vi "input.vi"(8 "error in":errorcluster, 10 "data table in":T1, 11 "FPGA Module runtime in":refnum<class "FPGA Module runtime.lvclass">) -> (0 "error out":errorcluster, 2 "data table out":T1, 3 "FPGA Module runtime out":refnum<class "FPGA Module runtime.lvclass">)   [LabVIEW 2014, in "FPGA Module runtime.lvclass"]
doc: "Provides an interface for reading data from a module at runtime. While this interface performs no operations, a child should provide an override which may read from any open sessions, references, or interfaces."
uses:
  FPGA Module runtime.lvclass
  <vilib>/NI/Tag Bus/table/data table.ctl
  FPGA Module runtime.lvclass/FPGA Module runtime.ctl
  OLD Project Folder/fpga channel/FXP I_20_5.ctl
  OLD Project Folder/fpga channel/FXP I_24_5.ctl
  OLD Project Folder/fpga channel/FXP I_24_10.ctl
  <vilib>/NI/Tag Bus/table/data polymorphs/write many/write Doubles.vi
  <vilib>/NI/Tag Bus/table/data polymorphs/write many/write Singles.vi
  <vilib>/NI/Tag Bus/table/data polymorphs/write many/write I64s.vi
  <vilib>/NI/Tag Bus/table/data polymorphs/write many/write I32s.vi
  <vilib>/NI/Tag Bus/table/data polymorphs/write many/write I16s.vi
  <vilib>/NI/Tag Bus/table/data polymorphs/write many/write I8s.vi
  <vilib>/NI/Tag Bus/table/data polymorphs/write many/write U64s.vi
  <vilib>/NI/Tag Bus/table/data polymorphs/write many/write U32s.vi
  <vilib>/NI/Tag Bus/table/data polymorphs/write many/write U16s.vi
  <vilib>/NI/Tag Bus/table/data polymorphs/write many/write U8s.vi
  <vilib>/NI/Tag Bus/table/data polymorphs/write many/write Booleans.vi
  <vilib>/NI/Tag Bus/table/data polymorphs/write one/write Array of Single.vi
  <vilib>/NI/Tag Bus/table/data polymorphs/write one/write Array of I64.vi
  <vilib>/NI/Tag Bus/table/data polymorphs/write one/write Array of I32.vi
  <vilib>/NI/Tag Bus/table/data polymorphs/write one/write Array of I16.vi
  <vilib>/NI/Tag Bus/table/data polymorphs/write one/write Array of I8.vi
  <vilib>/NI/Tag Bus/table/data polymorphs/write one/write Array of U64.vi
  <vilib>/NI/Tag Bus/table/data polymorphs/write one/write Array of U32.vi
  <vilib>/NI/Tag Bus/table/data polymorphs/write one/write Array of U16.vi
  <vilib>/NI/Tag Bus/table/data polymorphs/write one/write Array of U8.vi
  <vilib>/NI/Tag Bus/table/data polymorphs/write one/write Array of Boolean.vi
  <vilib>/rvi/errors/niLvFpgaAdjustHostInterfaceError.vi
  <vilib>/Utility/error.llb/Error Cluster From Error Code.vi
  <vilib>/rvi/interface/nirviReadWriteControl/nirviReadWriteControl.xnode
  <vilib>/NI/Tag Bus/table/data table.lvlib
  fpga channel/FPGA Channel.lvclass
  NiFpgaLv.dll
  <vilib>/rvi/interface/Simulation/niFpgaSimulationCallBeginRW.vi
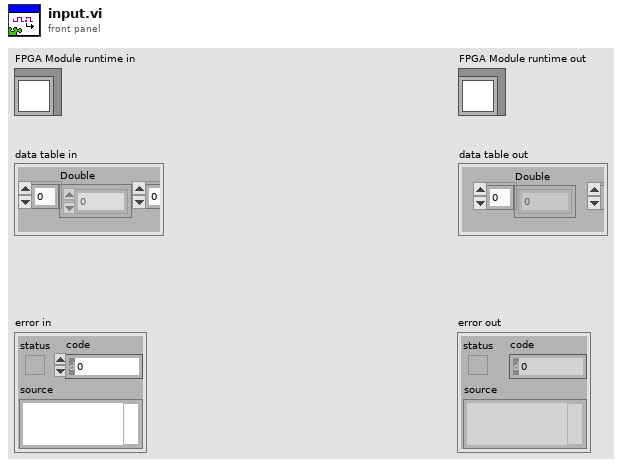
[diagram p1: front panel]
types:
  T1 = typedef "tag bus.lvlib/data table.lvlib/data table.ctl" = cluster{"Double":dbl[], "Single":sgl[], "I64":i64[], "I32":i32[], "I16":i16[], "I8":i8[], "U64":u64[], "U32":u32[], "U16":u16[], "U8":u8[], "Boolean":bool[], "String":string[], "Array of Double":cluster{"DBL Array":dbl[]}[], "Array of Single":cluster{"SGL Array":sgl[]}[], "Array of I64":cluster{"I64 Array":i64[]}[], "Array of I32":cluster{"I32 Array":i32[]}[], "Array of I16":cluster{"I16 Array":i16[]}[], "Array of I8":cluster{"I8 Array":i8[]}[], "Array of U64":cluster{"U64 Array":u64[]}[], "Array of U32":cluster{"U32 Array":u32[]}[], "Array of U16":cluster{"U16 Array":u16[]}[], "Array of U8":cluster{"U8 Array":u8[]}[], "Array of Boolean":cluster{"Boolean Array":bool[]}[], "Array of String":cluster{"String Array":string[]}[]}
  T2 = typedef "FPGA Module runtime.lvclass/ControlsMappings.ctl" = cluster{"data type":T3, "fpga res type":T4[], "fpga resource":refnum<k20>[], "data indexes":i32[]}
  T3 = typedef "tag bus.lvlib/tag descriptor.lvclass/Data Type.ctl" = enum16{"Double", "Single", "I64", "I32", "I16", "I8", "U64", "U32", "U16", "U8", "Boolean", "String", "Array of Double", "Array of Single", "Array of I64", "Array of I32", "Array of I16", "Array of I8", "Array of U64", "Array of U32", "Array of U16", "Array of U8", "Array of Boolean", "Array of String"}
  T4 = typedef "FPGA Channel.lvclass/fpga resource supported data types.ctl" = enum16{"Invalid Type", "Single", "I64", "I32", "I16", "I8", "U64", "U32", "U16", "U8", "Boolean", "FXP I,20,5", "FXP I,24,5", "FXP I,24,10", "Fifo 1023,I16"}
  T5 = typedef "FPGA Channel.lvclass/FXP I_20_5.ctl" = refnum<k20>
  T6 = typedef "FPGA Channel.lvclass/FXP I_24_5.ctl" = refnum<k20>
  T7 = typedef "FPGA Channel.lvclass/FXP I_24_10.ctl" = refnum<k20>
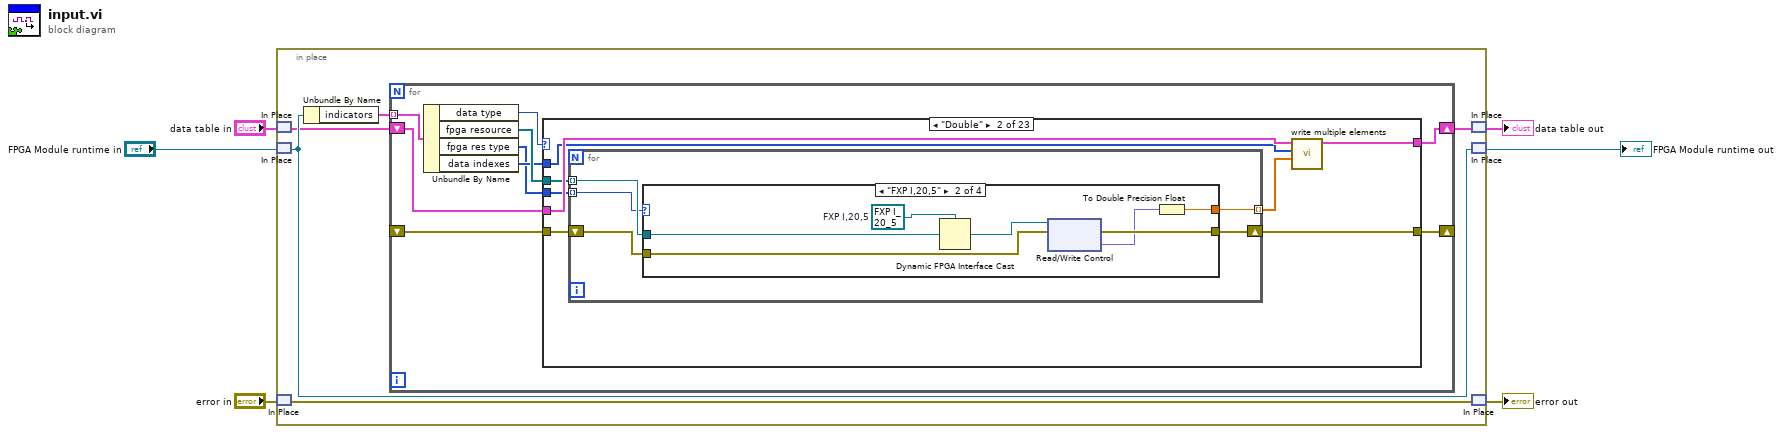
[diagram p0: block diagram]
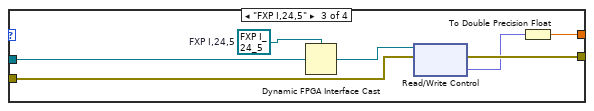
[diagram p4: hidden frame]
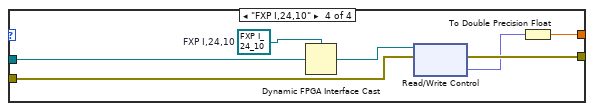
[diagram p5: hidden frame]
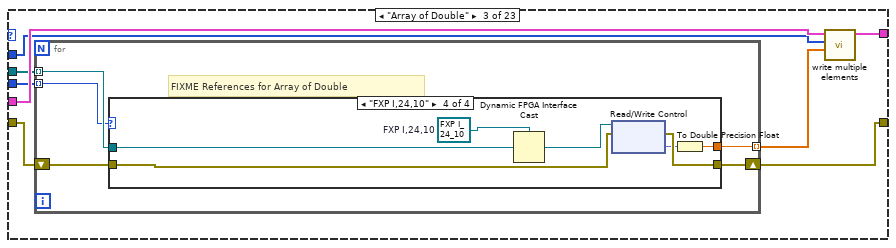
[diagram p6: hidden frame]
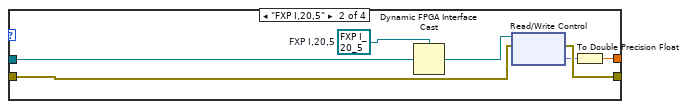
[diagram p8: hidden frame]
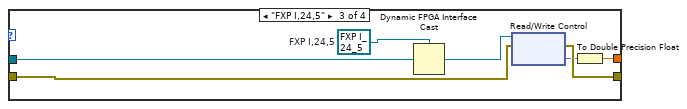
[diagram p9: hidden frame]
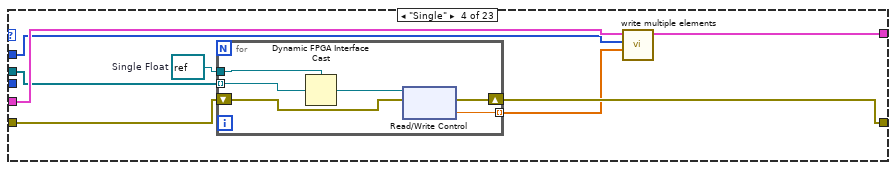
[diagram p10: hidden frame]
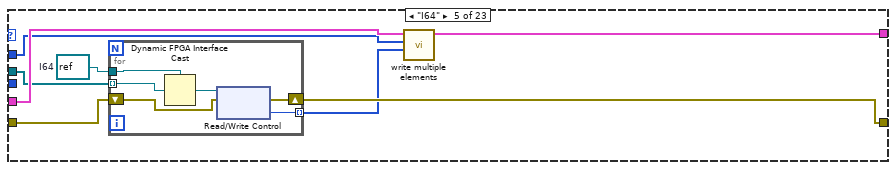
[diagram p11: hidden frame]
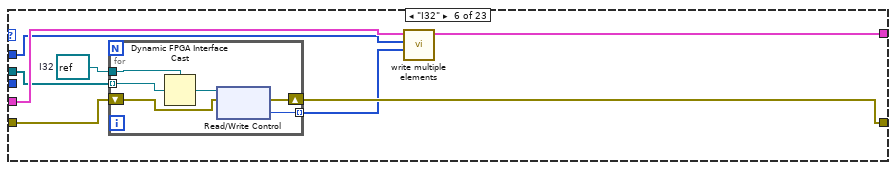
[diagram p12: hidden frame]
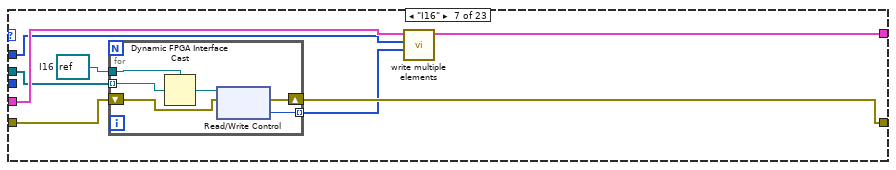
[diagram p13: hidden frame]
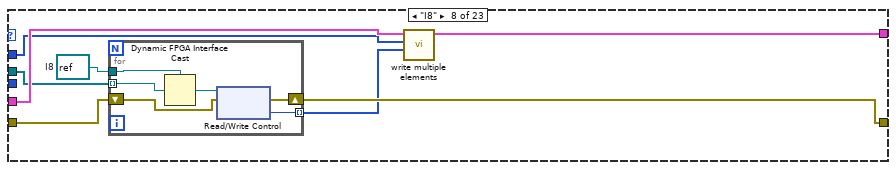
[diagram p14: hidden frame]
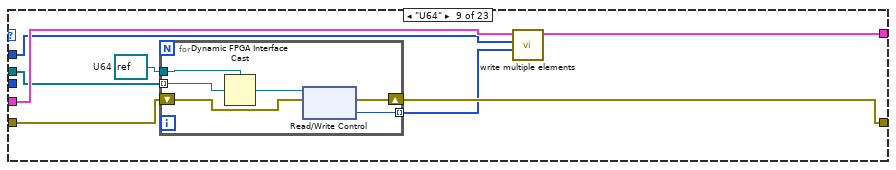
[diagram p15: hidden frame]
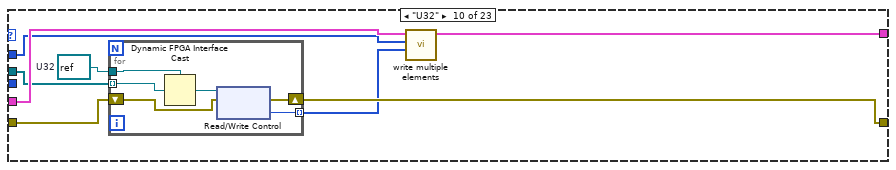
[diagram p16: hidden frame]
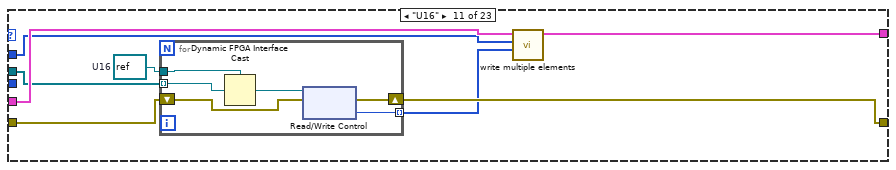
[diagram p17: hidden frame]
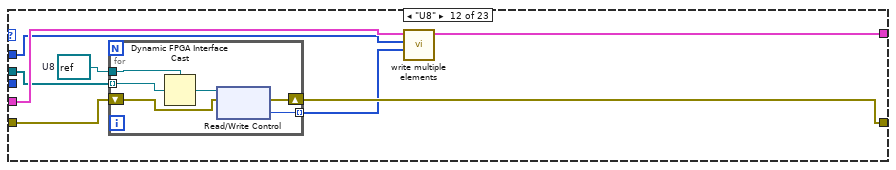
[diagram p18: hidden frame]
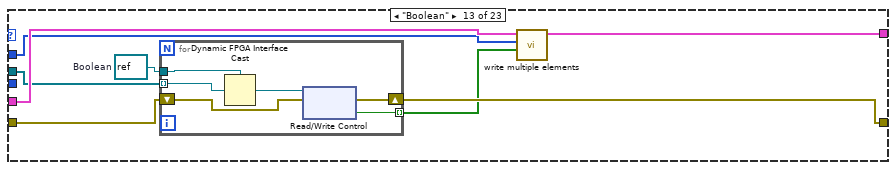
[diagram p19: hidden frame]
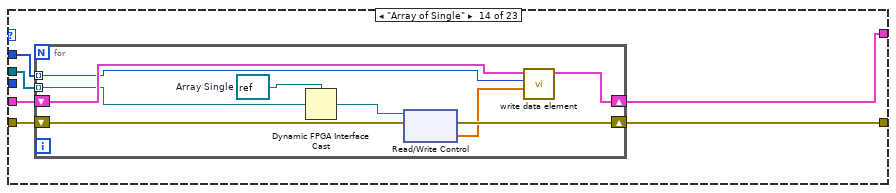
[diagram p20: hidden frame]
diagram:
  n1 = in-place {
    n2 = in-place-match #1("data table in") -> (w7:T1)
    n3 = in-place-match #2("FPGA Module runtime in") -> (w10:refnum<class "FPGA Module runtime.lvclass">)
    n4 = in-place-match #3("error in") -> (w11:errorcluster)
    n5 = Unbundle By Name(w10) -> ("indicators"=w8:T2[])
    n6 = for {
      shift-right: [w17] -> w9
      shift-left: w7 -> [w18]
      shift-right: [w16] -> _
      shift-left: _ -> [w15]
      tunnel: w8 -> [w20] mode=indexing
      n7 = Unbundle By Name(w20) -> ("data type"=w19:T3, "fpga resource"=w14:refnum<k20>[], "fpga res type"=w12:T4[], "data indexes"=w13:i32[])
      n8 = case shown="\"Double\"" w19 {
        tunnel: w13 -> [_ w23 w58 w98 w111 w126 w140 w154 w168 w182 w196 w210 w224 w236 w251 w266 w281 w296 w311 w326 w341 w356 w371]
        tunnel: w15 -> [w22 w27 w62 w96 w114 w124 w138 w152 w166 w180 w194 w208 w222 w235 w250 w265 w280 w295 w310 w325 w340 w355 w370]
        tunnel: w18 -> [w21 w30 w65 w100 w113 w128 w142 w156 w170 w184 w198 w212 w226 w238 w253 w268 w283 w298 w313 w328 w343 w358 w373]
        tunnel: [w21 w29 w64 w99 w112 w127 w141 w155 w169 w183 w197 w211 w225 w237 w252 w267 w282 w297 w312 w327 w342 w357 w372] -> w17
        tunnel: [w22 w26 w61 w95 w109 w123 w137 w151 w165 w179 w193 w207 w221 w234 w249 w264 w279 w294 w309 w324 w339 w354 w369] -> w16
        tunnel: w14 -> [_ w28 w63 w97 w110 w125 w139 w153 w167 w181 w195 w209 w223 w233 w248 w263 w278 w293 w308 w323 w338 w353 w368]
        tunnel: w12 -> [_ w25 w60 _ _ _ _ _ _ _ _ _ _ _ _ _ _ _ _ _ _ _ _]
        frame Default {
        }
        frame "Double" {
          n9 = for {
            tunnel: w28 -> [w35] mode=indexing
            shift-right: [w33] -> w26
            shift-left: w27 -> [w34]
            tunnel: [w32] -> w24 mode=indexing
            tunnel: w25 -> [w31] mode=indexing
            n10 = case shown="\"FXP I,20,5\"" w31 {
              tunnel: w35 -> [_ w43 w50 w57]
              tunnel: w34 -> [w36 w42 w49 w56]
              tunnel: [w36 w41 w48 w55] -> w33
              tunnel: [_ w38 w45 w52] -> w32
              frame "Invalid Type", Default {
              }
              frame "FXP I,20,5" {
                w40 = T5 refnum  # FXP I,20,5
                n11 = Dynamic FPGA Interface Cast(Session In=w40, Type=w43) -> (Session Out=w37:T5)
                n12 = xnode "Read/Write Control"("FPGA VI Reference In"=w37, "error in"=w42) -> ("error out"=w41:errorcluster, "Value"=w39:fxp<+/-,20,5>)  [unwired: 1 out]
                n13 = To Double Precision Float(number=w39) -> (double precision float=w38:dbl)
              }
              frame "FXP I,24,5" {
                w47 = T6 refnum  # FXP I,24,5
                n14 = Dynamic FPGA Interface Cast(Session In=w47, Type=w50) -> (Session Out=w44:T6)
                n15 = xnode "Read/Write Control"("FPGA VI Reference In"=w44, "error in"=w49) -> ("error out"=w48:errorcluster, "Value"=w46:fxp<+/-,24,5>)  [unwired: 1 out]
                n16 = To Double Precision Float(number=w46) -> (double precision float=w45:dbl)
              }
              frame "FXP I,24,10" {
                w54 = T7 refnum  # FXP I,24,10
                n17 = Dynamic FPGA Interface Cast(Session In=w54, Type=w57) -> (Session Out=w51:T7)
                n18 = xnode "Read/Write Control"("FPGA VI Reference In"=w51, "error in"=w56) -> ("error out"=w55:errorcluster, "Value"=w53:fxp<+/-,24,10>)  [unwired: 1 out]
                n19 = To Double Precision Float(number=w53) -> (double precision float=w52:dbl)
              }
            }
          }
          n20 = call-poly <vilib>:"write multiple elements.vi"("values"=w24, "indices"=w23, "data table in"=w30) -> ("data table out"=w29:T1)  [unwired: 8 in]
        }
        frame "Array of Double" {
          n21 = for {
            tunnel: w63 -> [w70] mode=indexing
            shift-right: [w68] -> w61
            shift-left: w62 -> [w69]
            tunnel: [w67] -> w59 mode=indexing
            tunnel: w60 -> [w66] mode=indexing
            # "FIXME References for Array of Double"
            n22 = case shown="\"FXP I,24,10\"" w66 {
              tunnel: w70 -> [_ w78 w85 w92]
              tunnel: w69 -> [w71 w77 w84 w91]
              tunnel: [w71 w76 w83 w90] -> w68
              tunnel: [_ w73 w80 w87] -> w67
              frame "Invalid Type", Default {
              }
              frame "FXP I,20,5" {
                w75 = T5 refnum  # FXP I,20,5
                n23 = Dynamic FPGA Interface Cast(Session In=w75, Type=w78) -> (Session Out=w72:T5)
                n24 = xnode "Read/Write Control"("FPGA VI Reference In"=w72, "error in"=w77) -> ("error out"=w76:errorcluster, "Value"=w74:fxp<+/-,20,5>)  [unwired: 1 out]
                n25 = To Double Precision Float(number=w74) -> (double precision float=w73:dbl)
              }
              frame "FXP I,24,5" {
                w82 = T6 refnum  # FXP I,24,5
                n26 = Dynamic FPGA Interface Cast(Session In=w82, Type=w85) -> (Session Out=w79:T6)
                n27 = xnode "Read/Write Control"("FPGA VI Reference In"=w79, "error in"=w84) -> ("error out"=w83:errorcluster, "Value"=w81:fxp<+/-,24,5>)  [unwired: 1 out]
                n28 = To Double Precision Float(number=w81) -> (double precision float=w80:dbl)
              }
              frame "FXP I,24,10" {
                w89 = T7 refnum  # FXP I,24,10
                n29 = Dynamic FPGA Interface Cast(Session In=w89, Type=w92) -> (Session Out=w86:T7)
                n30 = xnode "Read/Write Control"("FPGA VI Reference In"=w86, "error in"=w91) -> ("error out"=w90:errorcluster, "Value"=w88:fxp<+/-,24,10>)  [unwired: 1 out]
                n31 = To Double Precision Float(number=w88) -> (double precision float=w87:dbl)
              }
            }
          }
          n32 = call-poly <vilib>:"write multiple elements.vi"("values"=w59, "indices"=w58, "data table in"=w65) -> ("data table out"=w64:T1)  [unwired: 8 in]
        }
        frame "Single" {
          w94 = refnum<k20> refnum  # Single Float
          n33 = for {
            tunnel: w97 -> [w106] mode=indexing
            shift-right: [w103] -> w95
            shift-left: w96 -> [w104]
            tunnel: [w102] -> w93 mode=indexing
            tunnel: w94 -> [w101]
            n34 = Dynamic FPGA Interface Cast(Session In=w101, Type=w106) -> (Session Out=w105:refnum<k20>)
            n35 = xnode "Read/Write Control"("FPGA VI Reference In"=w105, "error in"=w104) -> ("error out"=w103:errorcluster, "Value"=w102:sgl)  [unwired: 1 out]
          }
          n36 = call-poly <vilib>:"write multiple elements.vi"("values"=w93, "indices"=w98, "data table in"=w100) -> ("data table out"=w99:T1)  [unwired: 8 in]
        }
        frame "I64" {
          w107 = refnum<k20> refnum  # I64
          n37 = for {
            tunnel: w110 -> [w120] mode=indexing
            shift-right: [w117] -> w109
            shift-left: w114 -> [w118]
            tunnel: [w116] -> w108 mode=indexing
            tunnel: w107 -> [w115]
            n38 = Dynamic FPGA Interface Cast(Session In=w115, Type=w120) -> (Session Out=w119:refnum<k20>)
            n39 = xnode "Read/Write Control"("FPGA VI Reference In"=w119, "error in"=w118) -> ("error out"=w117:errorcluster, "Value"=w116:i64)  [unwired: 1 out]
          }
          n40 = call-poly <vilib>:"write multiple elements.vi"("values"=w108, "indices"=w111, "data table in"=w113) -> ("data table out"=w112:T1)  [unwired: 8 in]
        }
        frame "I32" {
          w121 = refnum<k20> refnum  # I32
          n41 = for {
            tunnel: w125 -> [w134] mode=indexing
            shift-right: [w131] -> w123
            shift-left: w124 -> [w132]
            tunnel: [w130] -> w122 mode=indexing
            tunnel: w121 -> [w129]
            n42 = Dynamic FPGA Interface Cast(Session In=w129, Type=w134) -> (Session Out=w133:refnum<k20>)
            n43 = xnode "Read/Write Control"("FPGA VI Reference In"=w133, "error in"=w132) -> ("error out"=w131:errorcluster, "Value"=w130:i32)  [unwired: 1 out]
          }
          n44 = call-poly <vilib>:"write multiple elements.vi"("values"=w122, "indices"=w126, "data table in"=w128) -> ("data table out"=w127:T1)  [unwired: 8 in]
        }
        frame "I16" {
          w135 = refnum<k20> refnum  # I16
          n45 = for {
            tunnel: w139 -> [w148] mode=indexing
            shift-right: [w145] -> w137
            shift-left: w138 -> [w146]
            tunnel: [w144] -> w136 mode=indexing
            tunnel: w135 -> [w143]
            n46 = Dynamic FPGA Interface Cast(Session In=w143, Type=w148) -> (Session Out=w147:refnum<k20>)
            n47 = xnode "Read/Write Control"("FPGA VI Reference In"=w147, "error in"=w146) -> ("error out"=w145:errorcluster, "Value"=w144:i16)  [unwired: 1 out]
          }
          n48 = call-poly <vilib>:"write multiple elements.vi"("values"=w136, "indices"=w140, "data table in"=w142) -> ("data table out"=w141:T1)  [unwired: 8 in]
        }
        frame "I8" {
          w149 = refnum<k20> refnum  # I8
          n49 = for {
            tunnel: w153 -> [w162] mode=indexing
            shift-right: [w159] -> w151
            shift-left: w152 -> [w160]
            tunnel: [w158] -> w150 mode=indexing
            tunnel: w149 -> [w157]
            n50 = Dynamic FPGA Interface Cast(Session In=w157, Type=w162) -> (Session Out=w161:refnum<k20>)
            n51 = xnode "Read/Write Control"("FPGA VI Reference In"=w161, "error in"=w160) -> ("error out"=w159:errorcluster, "Value"=w158:i8)  [unwired: 1 out]
          }
          n52 = call-poly <vilib>:"write multiple elements.vi"("values"=w150, "indices"=w154, "data table in"=w156) -> ("data table out"=w155:T1)  [unwired: 8 in]
        }
        frame "U64" {
          w163 = refnum<k20> refnum  # U64
          n53 = for {
            tunnel: w167 -> [w176] mode=indexing
            shift-right: [w173] -> w165
            shift-left: w166 -> [w174]
            tunnel: [w172] -> w164 mode=indexing
            tunnel: w163 -> [w171]
            n54 = Dynamic FPGA Interface Cast(Session In=w171, Type=w176) -> (Session Out=w175:refnum<k20>)
            n55 = xnode "Read/Write Control"("FPGA VI Reference In"=w175, "error in"=w174) -> ("error out"=w173:errorcluster, "Value"=w172:u64)  [unwired: 1 out]
          }
          n56 = call-poly <vilib>:"write multiple elements.vi"("values"=w164, "indices"=w168, "data table in"=w170) -> ("data table out"=w169:T1)  [unwired: 8 in]
        }
        frame "U32" {
          w177 = refnum<k20> refnum  # U32
          n57 = for {
            tunnel: w181 -> [w190] mode=indexing
            shift-right: [w187] -> w179
            shift-left: w180 -> [w188]
            tunnel: [w186] -> w178 mode=indexing
            tunnel: w177 -> [w185]
            n58 = Dynamic FPGA Interface Cast(Session In=w185, Type=w190) -> (Session Out=w189:refnum<k20>)
            n59 = xnode "Read/Write Control"("FPGA VI Reference In"=w189, "error in"=w188) -> ("error out"=w187:errorcluster, "Value"=w186:u32)  [unwired: 1 out]
          }
          n60 = call-poly <vilib>:"write multiple elements.vi"("values"=w178, "indices"=w182, "data table in"=w184) -> ("data table out"=w183:T1)  [unwired: 8 in]
        }
        frame "U16" {
          w191 = refnum<k20> refnum  # U16
          n61 = for {
            tunnel: w195 -> [w204] mode=indexing
            shift-right: [w201] -> w193
            shift-left: w194 -> [w202]
            tunnel: [w200] -> w192 mode=indexing
            tunnel: w191 -> [w199]
            n62 = Dynamic FPGA Interface Cast(Session In=w199, Type=w204) -> (Session Out=w203:refnum<k20>)
            n63 = xnode "Read/Write Control"("FPGA VI Reference In"=w203, "error in"=w202) -> ("error out"=w201:errorcluster, "Value"=w200:u16)  [unwired: 1 out]
          }
          n64 = call-poly <vilib>:"write multiple elements.vi"("values"=w192, "indices"=w196, "data table in"=w198) -> ("data table out"=w197:T1)  [unwired: 8 in]
        }
        frame "U8" {
          w205 = refnum<k20> refnum  # U8
          n65 = for {
            tunnel: w209 -> [w218] mode=indexing
            shift-right: [w215] -> w207
            shift-left: w208 -> [w216]
            tunnel: [w214] -> w206 mode=indexing
            tunnel: w205 -> [w213]
            n66 = Dynamic FPGA Interface Cast(Session In=w213, Type=w218) -> (Session Out=w217:refnum<k20>)
            n67 = xnode "Read/Write Control"("FPGA VI Reference In"=w217, "error in"=w216) -> ("error out"=w215:errorcluster, "Value"=w214:u8)  [unwired: 1 out]
          }
          n68 = call-poly <vilib>:"write multiple elements.vi"("values"=w206, "indices"=w210, "data table in"=w212) -> ("data table out"=w211:T1)  [unwired: 8 in]
        }
        frame "Boolean" {
          w219 = refnum<k20> refnum  # Boolean
          n69 = for {
            tunnel: w223 -> [w232] mode=indexing
            shift-right: [w229] -> w221
            shift-left: w222 -> [w230]
            tunnel: [w228] -> w220 mode=indexing
            tunnel: w219 -> [w227]
            n70 = Dynamic FPGA Interface Cast(Session In=w227, Type=w232) -> (Session Out=w231:refnum<k20>)
            n71 = xnode "Read/Write Control"("FPGA VI Reference In"=w231, "error in"=w230) -> ("error out"=w229:errorcluster, "Value"=w228:bool)  [unwired: 1 out]
          }
          n72 = call-poly <vilib>:"write multiple elements.vi"("values"=w220, "indices"=w224, "data table in"=w226) -> ("data table out"=w225:T1)  [unwired: 8 in]
        }
        frame "Array of Single" {
          n73 = for {
            tunnel: w236 -> [w245] mode=indexing
            shift-right: [w242] -> w234
            shift-left: w235 -> [w241]
            shift-right: [w246] -> w237
            shift-left: w238 -> [w247]
            tunnel: w233 -> [w243] mode=indexing
            w240 = refnum<k20> refnum  # Array Single
            n74 = Dynamic FPGA Interface Cast(Session In=w240, Type=w243) -> (Session Out=w244:refnum<k20>)
            n75 = xnode "Read/Write Control"("FPGA VI Reference In"=w244, "error in"=w241) -> ("error out"=w242:errorcluster, "Value"=w239:sgl[])  [unwired: 1 out]
            n76 = call-poly <vilib>:"write data element.vi"("value"=w239, "index"=w245, "data table in"=w247) -> ("data table out"=w246:T1)  [unwired: 8 in]
          }
        }
        frame "Array of I64" {
          n77 = for {
            tunnel: w251 -> [w260] mode=indexing
            shift-right: [w257] -> w249
            shift-left: w250 -> [w256]
            shift-right: [w261] -> w252
            shift-left: w253 -> [w262]
            tunnel: w248 -> [w258] mode=indexing
            w254 = refnum<k20> refnum  # Array I64
            n78 = Dynamic FPGA Interface Cast(Session In=w254, Type=w258) -> (Session Out=w259:refnum<k20>)
            n79 = xnode "Read/Write Control"("FPGA VI Reference In"=w259, "error in"=w256) -> ("error out"=w257:errorcluster, "Value"=w255:i64[])  [unwired: 1 out]
            n80 = call-poly <vilib>:"write data element.vi"("value"=w255, "index"=w260, "data table in"=w262) -> ("data table out"=w261:T1)  [unwired: 8 in]
          }
        }
        frame "Array of I32" {
          n81 = for {
            tunnel: w266 -> [w275] mode=indexing
            shift-right: [w272] -> w264
            shift-left: w265 -> [w271]
            shift-right: [w276] -> w267
            shift-left: w268 -> [w277]
            tunnel: w263 -> [w273] mode=indexing
            w269 = refnum<k20> refnum  # Array I32
            n82 = Dynamic FPGA Interface Cast(Session In=w269, Type=w273) -> (Session Out=w274:refnum<k20>)
            n83 = xnode "Read/Write Control"("FPGA VI Reference In"=w274, "error in"=w271) -> ("error out"=w272:errorcluster, "Value"=w270:i32[])  [unwired: 1 out]
            n84 = call-poly <vilib>:"write data element.vi"("value"=w270, "index"=w275, "data table in"=w277) -> ("data table out"=w276:T1)  [unwired: 8 in]
          }
        }
        frame "Array of I16" {
          n85 = for {
            tunnel: w281 -> [w290] mode=indexing
            shift-right: [w287] -> w279
            shift-left: w280 -> [w286]
            shift-right: [w291] -> w282
            shift-left: w283 -> [w292]
            tunnel: w278 -> [w288] mode=indexing
            w284 = refnum<k20> refnum  # Array I16
            n86 = Dynamic FPGA Interface Cast(Session In=w284, Type=w288) -> (Session Out=w289:refnum<k20>)
            n87 = xnode "Read/Write Control"("FPGA VI Reference In"=w289, "error in"=w286) -> ("error out"=w287:errorcluster, "Value"=w285:i16[])  [unwired: 1 out]
            n88 = call-poly <vilib>:"write data element.vi"("value"=w285, "index"=w290, "data table in"=w292) -> ("data table out"=w291:T1)  [unwired: 8 in]
          }
        }
        frame "Array of I8" {
          n89 = for {
            tunnel: w296 -> [w305] mode=indexing
            shift-right: [w302] -> w294
            shift-left: w295 -> [w301]
            shift-right: [w306] -> w297
            shift-left: w298 -> [w307]
            tunnel: w293 -> [w303] mode=indexing
            w299 = refnum<k20> refnum  # Array I8
            n90 = Dynamic FPGA Interface Cast(Session In=w299, Type=w303) -> (Session Out=w304:refnum<k20>)
            n91 = xnode "Read/Write Control"("FPGA VI Reference In"=w304, "error in"=w301) -> ("error out"=w302:errorcluster, "Value"=w300:i8[])  [unwired: 1 out]
            n92 = call-poly <vilib>:"write data element.vi"("value"=w300, "index"=w305, "data table in"=w307) -> ("data table out"=w306:T1)  [unwired: 8 in]
          }
        }
        frame "Array of U64" {
          n93 = for {
            tunnel: w311 -> [w320] mode=indexing
            shift-right: [w317] -> w309
            shift-left: w310 -> [w316]
            shift-right: [w321] -> w312
            shift-left: w313 -> [w322]
            tunnel: w308 -> [w318] mode=indexing
            n94 = Dynamic FPGA Interface Cast(Session In=refnum<k20> refnum ("FPGA VI Reference Out"), Type=w318) -> (Session Out=w319:refnum<k20>)
            n95 = xnode "Read/Write Control"("FPGA VI Reference In"=w319, "error in"=w316) -> ("error out"=w317:errorcluster, "Value"=w315:u64[])  [unwired: 1 out]
            n96 = call-poly <vilib>:"write data element.vi"("value"=w315, "index"=w320, "data table in"=w322) -> ("data table out"=w321:T1)  [unwired: 8 in]
          }
        }
        frame "Array of U32" {
          n97 = for {
            tunnel: w326 -> [w335] mode=indexing
            shift-right: [w332] -> w324
            shift-left: w325 -> [w331]
            shift-right: [w336] -> w327
            shift-left: w328 -> [w337]
            tunnel: w323 -> [w333] mode=indexing
            w329 = refnum<k20> refnum  # Array U32
            n98 = Dynamic FPGA Interface Cast(Session In=w329, Type=w333) -> (Session Out=w334:refnum<k20>)
            n99 = xnode "Read/Write Control"("FPGA VI Reference In"=w334, "error in"=w331) -> ("error out"=w332:errorcluster, "Value"=w330:u32[])  [unwired: 1 out]
            n100 = call-poly <vilib>:"write data element.vi"("value"=w330, "index"=w335, "data table in"=w337) -> ("data table out"=w336:T1)  [unwired: 8 in]
          }
        }
        frame "Array of U16" {
          n101 = for {
            tunnel: w341 -> [w350] mode=indexing
            shift-right: [w347] -> w339
            shift-left: w340 -> [w346]
            shift-right: [w351] -> w342
            shift-left: w343 -> [w352]
            tunnel: w338 -> [w348] mode=indexing
            w344 = refnum<k20> refnum  # Array U16
            n102 = Dynamic FPGA Interface Cast(Session In=w344, Type=w348) -> (Session Out=w349:refnum<k20>)
            n103 = xnode "Read/Write Control"("FPGA VI Reference In"=w349, "error in"=w346) -> ("error out"=w347:errorcluster, "Value"=w345:u16[])  [unwired: 1 out]
            n104 = call-poly <vilib>:"write data element.vi"("value"=w345, "index"=w350, "data table in"=w352) -> ("data table out"=w351:T1)  [unwired: 8 in]
          }
        }
        frame "Array of U8" {
          n105 = for {
            tunnel: w356 -> [w365] mode=indexing
            shift-right: [w362] -> w354
            shift-left: w355 -> [w361]
            shift-right: [w366] -> w357
            shift-left: w358 -> [w367]
            tunnel: w353 -> [w363] mode=indexing
            w359 = refnum<k20> refnum  # Array U8
            n106 = Dynamic FPGA Interface Cast(Session In=w359, Type=w363) -> (Session Out=w364:refnum<k20>)
            n107 = xnode "Read/Write Control"("FPGA VI Reference In"=w364, "error in"=w361) -> ("error out"=w362:errorcluster, "Value"=w360:u8[])  [unwired: 1 out]
            n108 = call-poly <vilib>:"write data element.vi"("value"=w360, "index"=w365, "data table in"=w367) -> ("data table out"=w366:T1)  [unwired: 8 in]
          }
        }
        frame "Array of Boolean" {
          n109 = for {
            tunnel: w371 -> [w380] mode=indexing
            shift-right: [w377] -> w369
            shift-left: w370 -> [w376]
            shift-right: [w381] -> w372
            shift-left: w373 -> [w382]
            tunnel: w368 -> [w378] mode=indexing
            w374 = refnum<k20> refnum  # Array Boolean
            n110 = Dynamic FPGA Interface Cast(Session In=w374, Type=w378) -> (Session Out=w379:refnum<k20>)
            n111 = xnode "Read/Write Control"("FPGA VI Reference In"=w379, "error in"=w376) -> ("error out"=w377:errorcluster, "Value"=w375:bool[])  [unwired: 1 out]
            n112 = call-poly <vilib>:"write data element.vi"("value"=w375, "index"=w380, "data table in"=w382) -> ("data table out"=w381:T1)  [unwired: 8 in]
          }
        }
      }
    }
    n113 = in-place-match #1(w9) -> (→"data table out":T1)
    n114 = in-place-match #2(w10) -> (→"FPGA Module runtime out":refnum<class "FPGA Module runtime.lvclass">)
    n115 = in-place-match #3(w11) -> (→"error out":errorcluster)
  }
